vi "Teardown.vi"(8 "Error in":errorcluster, 11 "Project Stuff in":refnum<class "Project Stuff.lvclass">) -> (0 "Error out":errorcluster)   [LabVIEW 2020, in "_Shared.lvlib" / "Project Stuff.lvclass"]
uses:
  Project Stuff.lvclass
  Project Stuff.lvclass/Project Stuff.ctl
  <vilib>/Utility/EditLVProj/Edit LVProj.lvlib
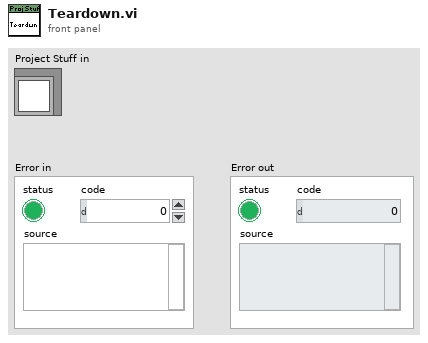
[diagram p1: front panel]
types:
  T1 = typedef "Edit LVProj.lvlib/Library And VI References.ctl" = cluster{"Target Reference":refnum<vi>, "VI References":refnum<vi>[], "Library References":refnum<vi>[]}
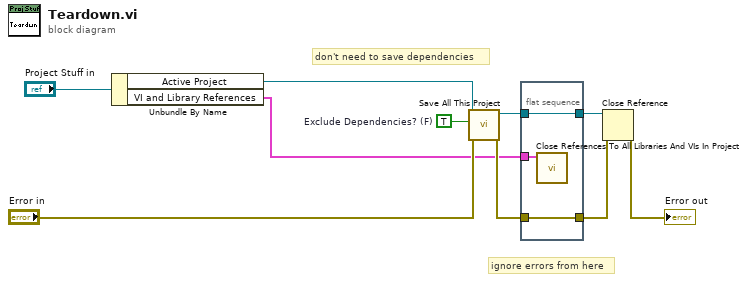
[diagram p0: block diagram]
diagram:
  w8 = TRUE  # Exclude Dependencies? (F)
  # "don't need to save dependencies"
  # "ignore errors from here"
  n1 = Unbundle By Name("Project Stuff in") -> ("Active Project"=w4:refnum<vi>, "VI and Library References"=w3:T1[])
  n2 = call <vilib>:"Save All This Project.vi"("error in (no error)"="Error in", "Exclude Dependencies? (F)"=w8, "Project in"=w4) -> ("error out"=w9:errorcluster, "Project out"=w1:refnum<vi>)  [unwired: 7 in]
  n3 = flat-sequence {
    tunnel: [w11] -> w10
    tunnel: w9 -> [w11]
    tunnel: w3 -> [w13]
    tunnel: [w12] -> w2
    tunnel: w1 -> [w12]
    frame #0 {
      n4 = call <vilib>:"Close References To All Libraries And VIs In Project.vi"("VI and Library References"=w13) -> ()  [unwired: 10 in, 1 out]
    }
  }
  n5 = Close Reference(reference=w2, error in (no error)=w10) -> (error out=→"Error out":errorcluster)
